vi "ErdosBorwein.vi"() -> (0 "Erdós-Borwein constant":ext format="%_15f")   [LabVIEW 2017, in "GPNumeric.lvlib"]
doc: "This constant is inlined.\n\nSteen Schmidt\nGPower\n12/1 2015"
uses:
  GPNumeric.lvlib
panel:
  # "Copyright © 2015\nGPower\nSee enclosed license file for terms and conditions"
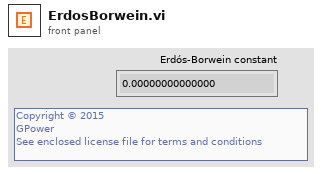
[diagram p1: front panel]
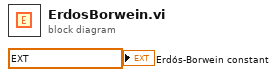
[diagram p0: block diagram]
diagram:
  "Erdós-Borwein constant" <- ext 1.60669515241529176
